vi "read-PLT-inkscape.vi"() -> ()   [LabVIEW 2014]
doc: "André Romero - 2016\nandretec@ifsc.usp.br\n\nRead PLT files and convert in coordenates"
panel:
  out "Pen":bool[](array[boolean])
  out "Y":ext[](array[numeric])
  out "X":ext[](array[numeric])
  in  "file path (dialog if empty)":path=path "C:/Documents and Settings/NI-Vision/Desktop/DecodeX/ink-1.plt"
  out "output 1":string="PD"
  out "output 2":i32=5344
  out "output 3":i32=8289
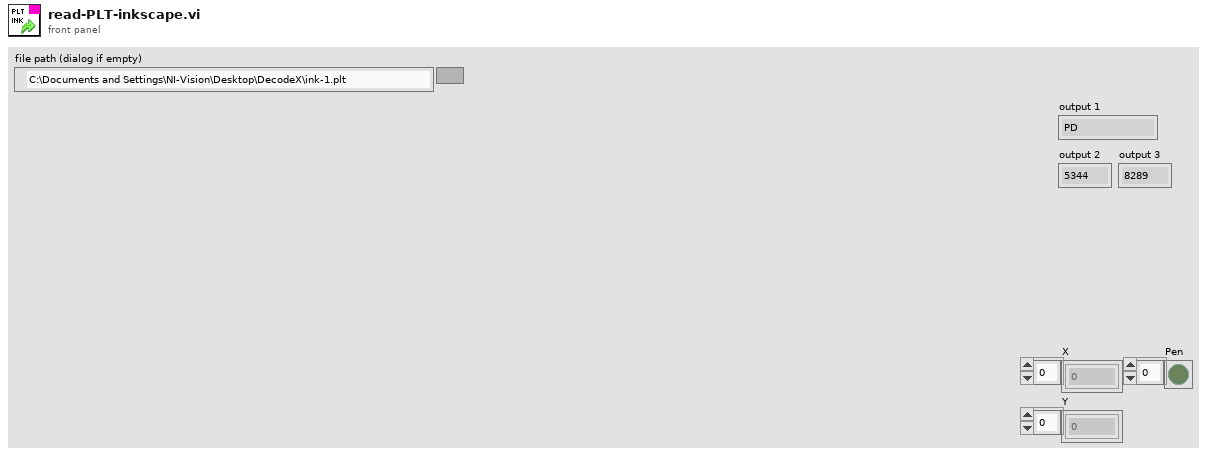
[diagram p1: front panel]
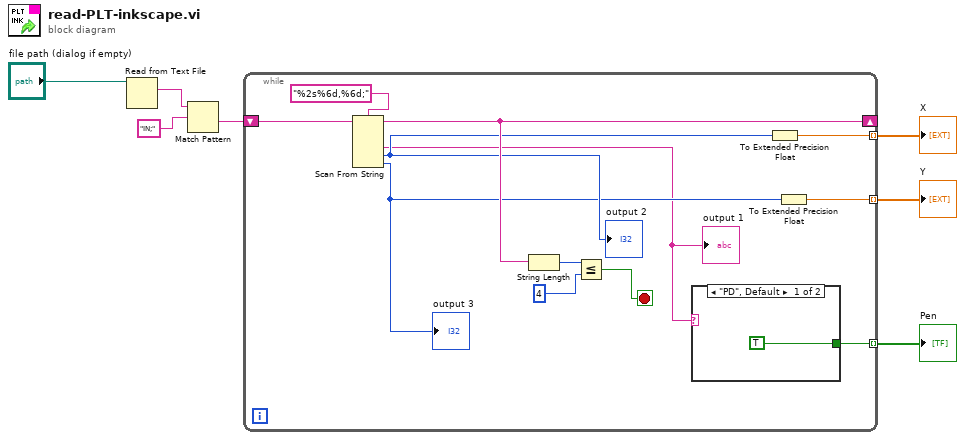
[diagram p0: block diagram]
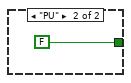
[diagram p2: hidden frame]
diagram:
  n1 = Read from Text File(file (use dialog)="file path (dialog if empty)") -> (text=w6:string)  [unwired: 3 in, 3 out]
  n2 = Match Pattern(string=w6, regular expression="IN;") -> (after substring=w4:string)  [unwired: 1 in, 3 out]
  n3 = while {
    shift-right: [w17] -> _
    shift-left: w4 -> [w18]
    tunnel: [w9] -> w3 mode=indexing
    tunnel: [w8] -> w2 mode=indexing
    tunnel: [w10] -> w1 mode=indexing
    stop <- w14 stop-if-true
    n4 = Scan From String(format string="%2s%6d,%6d;", input string=w18) -> (remaining string=w17:string, output 1=w11:string, output 2=w13:i32, output 3=w12:i32)  [unwired: 5 in, 2 out]
    "output 1" <- w11
    "output 2" <- w13
    "output 3" <- w12
    n5 = String Length(string=w17) -> (length=w16:i32)
    n6 = Less Or Equal?(x=w16, y=4) -> (x <= y?=w14:bool)
    n7 = case shown="\"PD\", Default" w11 {
      tunnel: [TRUE FALSE] -> w10
      frame "PD", Default {
      }
      frame "PU" {
      }
    }
    n8 = To Extended Precision Float(1:w13) -> (0:w9:ext)
    n9 = To Extended Precision Float(1:w12) -> (0:w8:ext)
  }
  "X" <- w3
  "Y" <- w2
  "Pen" <- w1
